vi "Packetize.vi"(0 "Arduino Resource":T1={"VISA resource"="", "Board Type"=enum."Uno", "Connection Type"=enum."USB / Serial", "Bytes Per Packet (15)"=15}, 7 "Data":u8[](array[numeric]), 11 "error in":errorcluster) -> (4 "Arduino Resource":T1={"VISA resource"="", "Board Type"=enum."Uno", "Connection Type"=enum."USB / Serial", "Bytes Per Packet (15)"=15}, 8 "Packet":string, 15 "error out":errorcluster)   [LabVIEW 2015, in "LabVIEW Interface for Arduino.lvlib"]
doc: "Pack data into packets including checksum and ensure fixed packet length."
uses:
  <vilib>/LabVIEW Interface for Arduino/LabVIEW Interface for Arduino.lvlib
  <vilib>/LabVIEW Interface for Arduino/Type Defs/Arduino Resource.ctl
  <vilib>/LabVIEW Interface for Arduino/Type Defs/Board Type.ctl
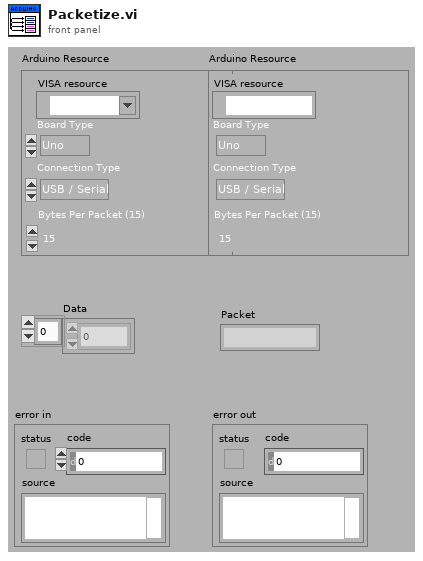
[diagram p1: front panel]
types:
  T1 = typedef "LabVIEW Interface for Arduino.lvlib/Arduino Resource.ctl" = cluster{"VISA resource":refnum<visa-resource-name>, "Board Type":T2, "Connection Type":enum8{"USB / Serial"}, "Bytes Per Packet (15)":u8}
  T2 = typedef "LabVIEW Interface for Arduino.lvlib/Board Type.ctl" = enum16{"Uno", "Dimuelanove w/Atmega 328", "Mega 2560"}
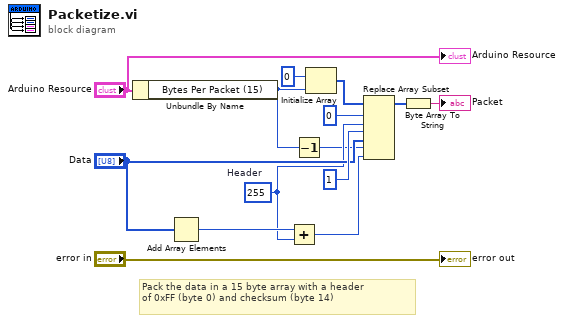
[diagram p0: block diagram]
diagram:
  w7 = u8 255  # Header
  # "Pack the data in a 15 byte array with a header \nof 0xFF (byte 0) and checksum (byte 14)"
  n1 = Unbundle By Name("Arduino Resource") -> ("Bytes Per Packet (15)"=w3:u8)
  n2 = Add Array Elements(numeric array="Data") -> (sum=w8:u8)
  n3 = Add(x=w8, y=w7) -> (x+y=w6:u8)
  n4 = Decrement(x=w3) -> (x-1=w4:u8)
  n5 = Initialize Array(u8 0, w3) -> (w14:u8[])
  n6 = Replace Array Subset(array=w14, new element #1=w7, index #1=0 ("index"), new element #2="Data", index #2=1 ("index"), new element #3=w6, index #3=w4) -> (w5:u8[])
  n7 = Byte Array To String(unsigned byte array=w5) -> (string=→"Packet":string)
  "Arduino Resource" <- "Arduino Resource"
  "error out" <- "error in"
